vi "10_NOV_VARY_V_filtered_I.vi"() -> ()   [LabVIEW 2020]
uses:
  <instrlib>/Agilent B2900 Series/Agilent B2900 Series.lvlib
  <vilib>/ptbypt/NI_PtbyPt.lvlib
panel:
  in  "Filter":bool=TRUE
  in  "Voltage(V)":dbl(slide) scale=0.0..0.1
  out "Measured Current (Amp)":dbl
  in  "Stop Button":bool
  out "Waveform Chart":dbl(graph)
  in  "SELECT DEVICE":refnum<visa-resource-name>="USB0::0x0957::0x8E18::MY51140695::INSTR"
  in  "Channel":enum16{"Not Selected", "1", "2"}(ring)
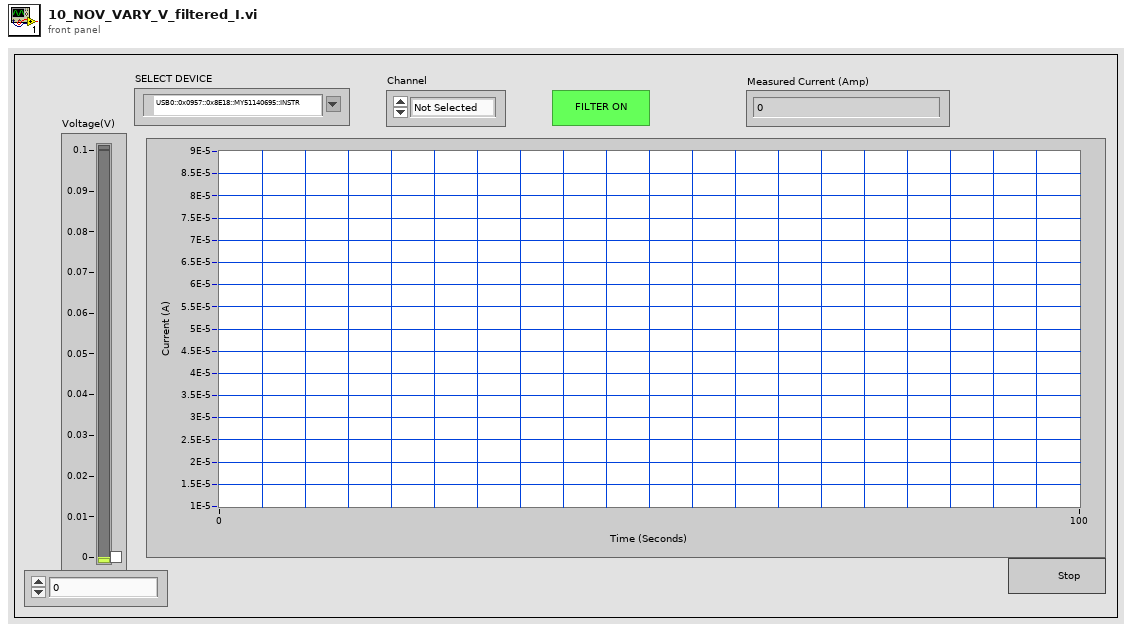
[diagram p1: front panel]
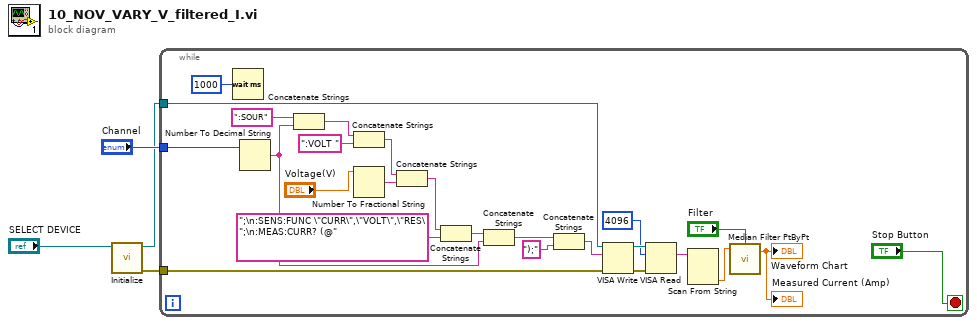
[diagram p0: block diagram]
diagram:
  n1 = call <instrlib>:"Initialize.vi"("VISA resource name"="SELECT DEVICE") -> ("error out"=w1:errorcluster, "VISA resource name out"=w2:refnum<visa-resource-name>)  [unwired: 9 in]
  n2 = while {
    tunnel: "Channel" -> [w27]
    tunnel: w2 -> [w16]
    tunnel: w1 -> [w15]
    stop <- "Stop Button" stop-if-true
    n3 = Wait (ms)(milliseconds to wait=u32 1000) -> ()  [unwired: 1 out]
    n4 = Number To Decimal String(number=w27) -> (decimal integer string=w20:string)  [unwired: 1 in]
    n5 = Concatenate Strings(":SOUR", w20) -> (w19:string)
    n6 = Concatenate Strings(w19, ":VOLT ") -> (w17:string)
    n7 = Number To Fractional String(number="Voltage(V)") -> (F-format string=w28:string)  [unwired: 3 in]
    n8 = Concatenate Strings(w17, w28) -> (w26:string)
    n9 = Concatenate Strings(w26, ";\n:SENS:FUNC \"CURR\",\"VOLT\",\"RES\";\n:MEAS:CURR? (@") -> (w24:string)
    n10 = Concatenate Strings(w24, w20) -> (w23:string)
    n11 = Concatenate Strings(w23, ");" ("string")) -> (w14:string)
    n12 = VISA Write(VISA resource name=w16, write buffer=w14, error in (no error)=w15) -> (VISA resource name out=w13:refnum<visa-resource-name>, error out=w12:errorcluster)  [unwired: 1 out]
    n13 = VISA Read(VISA resource name=w13, byte count=u32 4096, error in (no error)=w12) -> (read buffer=w8:string)  [unwired: 3 out]
    n14 = Scan From String(input string=w8) -> (output 1=w6:dbl)  [unwired: 4 in, 3 out]
    n15 = call <vilib>:"Median Filter PtByPt.vi"("initialize"="Filter", "x"=w6) -> ("Filtered x"=→"Measured Current (Amp)" →"Waveform Chart":dbl)  [unwired: 2 in, 1 out]
  }
